vi "test14-Interrupt_Event.vi"(8 "error in (no error)":errorcluster, 11 "TestCase in":refnum<class "testcase-CSMGlobalLog.lvclass">) -> (0 "error out":errorcluster, 3 "TestCase out":refnum<class "testcase-CSMGlobalLog.lvclass">)   [LabVIEW 2017, in "testcase-CSMGlobalLog.lvclass"]
uses:
  testcase-CSMGlobalLog.lvclass
  testcase-CSMGlobalLog.lvclass/testcase-CSMGlobalLog.ctl
  src/user.lib/_NEVSTOP/Communicable State Machine(CSM)/_Support/Typedef/_CSM_GlobalLog_MSG.ctl
  src/user.lib/_NEVSTOP/Communicable State Machine(CSM)/_Support/Typedef/_CSM_Response Source Message.ctl
  src/user.lib/_NEVSTOP/Communicable State Machine(CSM)/_Support/Typedef/_CSM_GlobalLog_MSG_TYPE.ctl
  c0dc643a-0362-49fc-99f4-5251266ba5a0.vi
  src/user.lib/_NEVSTOP/Communicable State Machine(CSM)/_Support/GlobalEvent/GEvt-Generate with Rule Check.vi
  src/user.lib/_NEVSTOP/Communicable State Machine(CSM)/AdvanceAPI/CSM - Convert Error to Argument.vi
  src/user.lib/_NEVSTOP/Communicable State Machine(CSM)/AdvanceAPI/CSM - Make String Arguments Safe.vi
  src/user.lib/_NEVSTOP/Communicable State Machine(CSM)/AdvanceAPI/CSM - Keywords.vi
  src/user.lib/_NEVSTOP/Communicable State Machine(CSM)/_Support/GlobalEvent/Cache-GEvt Refs.vi
  src/user.lib/_NEVSTOP/Communicable State Machine(CSM)/_Support/GlobalEvent/LogFilter/LogFilter - Check.vi
  src/user.lib/_NEVSTOP/Communicable State Machine(CSM)/_Support/GlobalEvent/LogFilter/LogFilter.lvclass
  <vilib>/addons/_JKI Toolkits/VI Tester/TestCase.llb/TestCase.lvclass
  src/user.lib/_NEVSTOP/Communicable State Machine(CSM)/Communicable State Machine.lvlib
  C:/Program Files (x86)/National Instruments/LabVIEW 2017/vi.lib/addons/_JKI Toolkits/VI Tester/TestCase.llb/TestCase.lvclass
panel:
  out "String cache each loop":string
  out "error out 2":errorcluster
  out "Timed out":bool[](array[boolean])
  out "LoopCount":i32
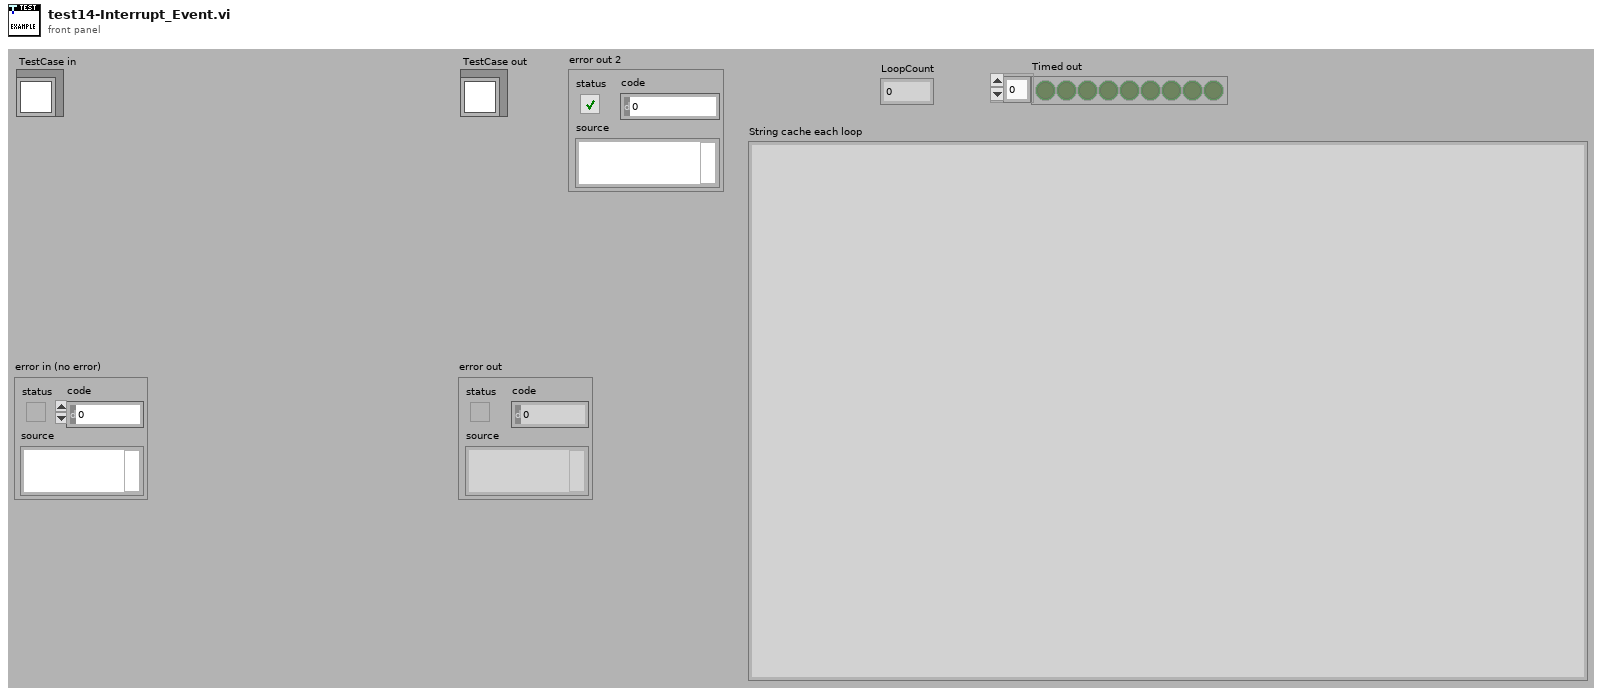
[diagram p1: front panel]
types:
  T1 = typedef "Communicable State Machine.lvlib/_CSM_GlobalLog_MSG.ctl" = cluster{"Name (\"\" to Use UUID)":string, "Current State":string, "Arguments":string, "Source Message":T2, "Source Module":string, "Complete(T)/Start(F)":bool, "LogType":T3, "Time Stamp":timestamp}
  T2 = typedef "Communicable State Machine.lvlib/_CSM_Response Source Message.ctl" = cluster{"‘State":string, "’Arguments":string, "’Error":errorcluster}
  T3 = typedef "Communicable State Machine.lvlib/_CSM_GlobalLog_MSG_TYPE.ctl" = enum16{"User Log", "State Change", "Status", "Interrupt", "Register", "Unregister", "Error Log", "Module Created", "Module Destroyed", "Async Message", "No-Rep Async Message", "Sync Message"}
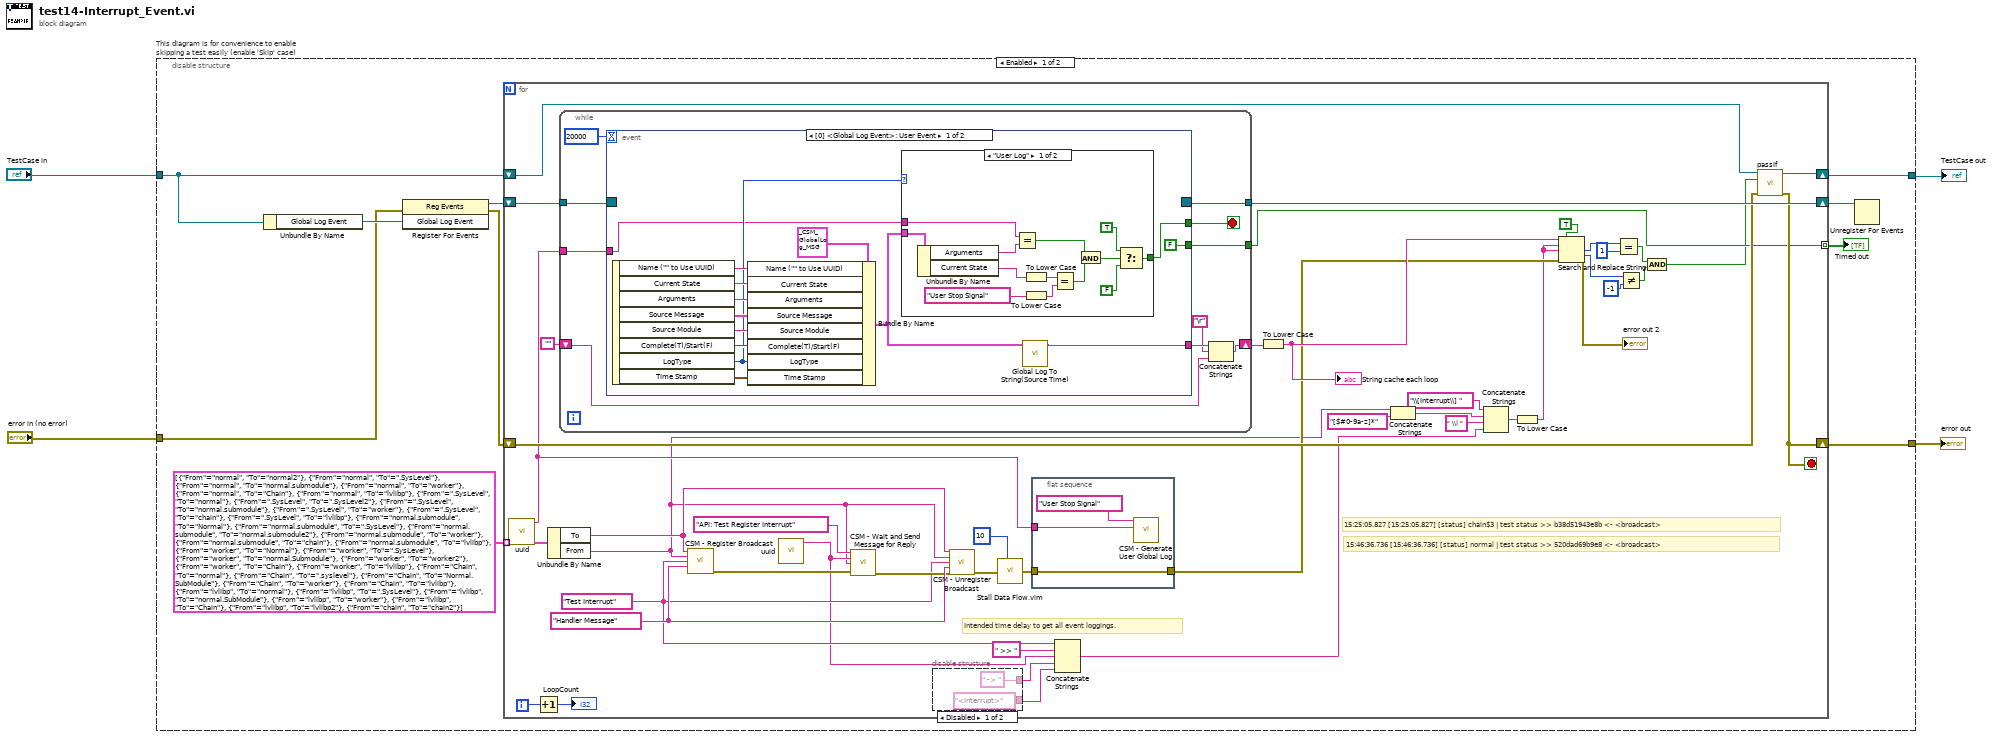
[diagram p0: block diagram]
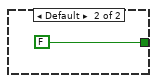
[diagram p3: hidden frame]
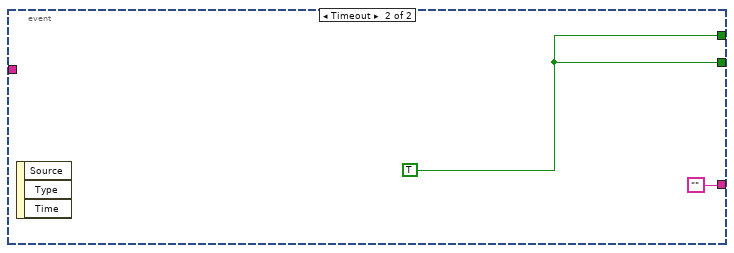
[diagram p4: hidden frame]
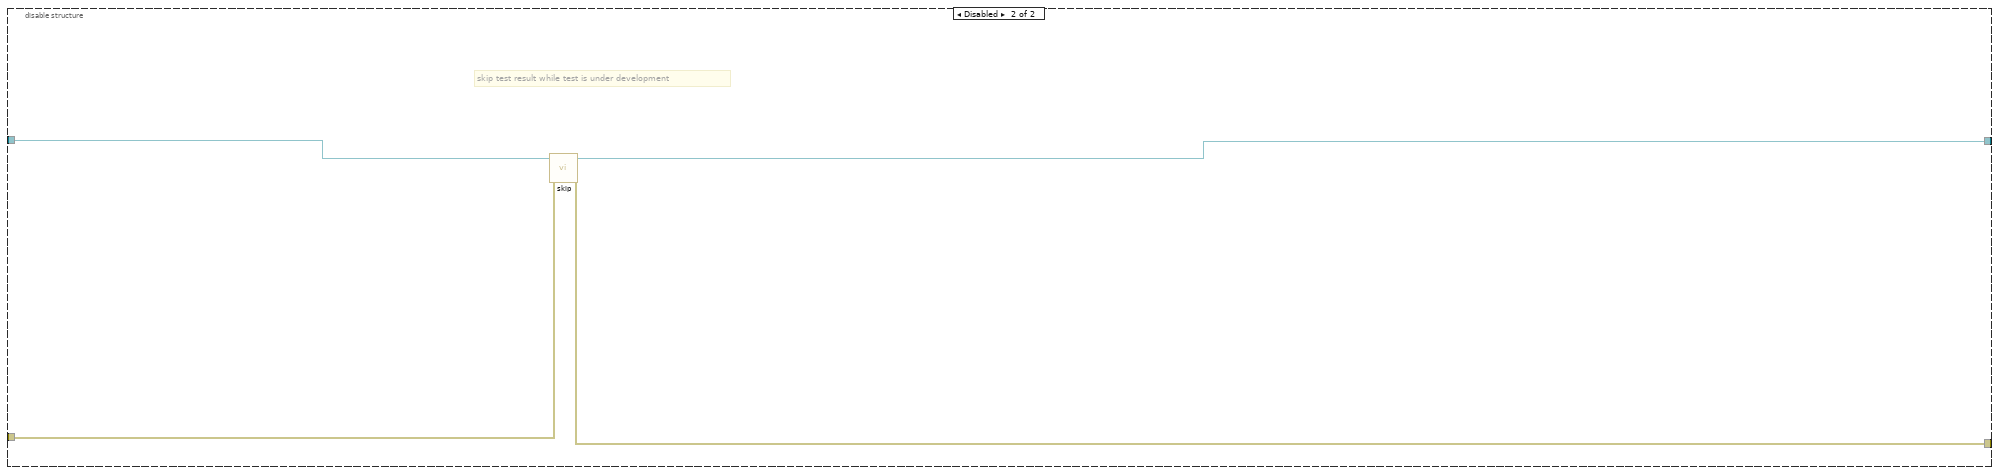
[diagram p5: hidden frame]
diagram:
  n1 = disable-structure "This diagram is for convenience to enable skipping a test easily (enable 'Skip' case)" shown="Enabled" {
    disable-tunnel: "TestCase in" -> [w9 w108]
    disable-tunnel: [w8 w106] -> w1
    disable-tunnel: [w7 w107] -> w3
    disable-tunnel: "error in (no error)" -> [w13 w105]
    frame Enabled {
      n2 = Unbundle By Name(w9) -> ("Global Log Event"=w14:refnum<user-event>)
      n3 = register-events(error in=w13, w14) -> (reference out=w12:refnum<event-registration>, error out=w10:errorcluster)  [unwired: 1 in]
      n4 = for {
        shift-right: [w58] -> w11
        shift-left: w12 -> [w59]
        shift-right: [w54] -> w7
        shift-left: w10 -> [w56]
        tunnel: cluster{"From":string, "To":string}[] [{"From"="normal", "To"="normal2"}, {"From"="normal", "To"=".SysLevel"}, {"From"="normal", "To"="normal.submodule"}, {"From"="normal", "To"="worker"}, {"From"="normal", "To"="Chain"}, {"From"="normal", "To"="lvlibp"}, {"From"=".SysLevel", "To"="normal"}, {"From"=".SysLevel", "To"=".SysLevel2"}, {"From"=".SysLevel", "To"="normal.submodule"}, {"From"=".SysLevel", "To"="worker"}, {"From"=".SysLevel", "To"="chain"}, {"From"=".SysLevel", "To"="lvlibp"}, {"From"="normal.submodule", "To"="Normal"}, {"From"="normal.submodule", "To"=".SysLevel"}, {"From"="normal.submodule", "To"="normal.submodule2"}, {"From"="normal.submodule", "To"="worker"}, {"From"="normal.submodule", "To"="chain"}, {"From"="normal.submodule", "To"="lvlibp"}, {"From"="worker", "To"="Normal"}, {"From"="worker", "To"=".SysLevel"}, {"From"="worker", "To"="normal.Submodule"}, {"From"="worker", "To"="worker2"}, {"From"="worker", "To"="Chain"}, {"From"="worker", "To"="lvlibp"}, {"From"="Chain", "To"="normal"}, {"From"="Chain", "To"=".syslevel"}, {"From"="Chain", "To"="Normal.SubModule"}, {"From"="Chain", "To"="worker"}, {"From"="Chain", "To"="lvlibp"}, {"From"="lvlibp", "To"="normal"}, {"From"="lvlibp", "To"=".SysLevel"}, {"From"="lvlibp", "To"="normal.SubModule"}, {"From"="lvlibp", "To"="worker"}, {"From"="lvlibp", "To"="Chain"}, {"From"="lvlibp", "To"="lvlibp2"}, {"From"="chain", "To"="chain2"}] -> [w31] mode=indexing
        shift-right: [w57] -> w8
        shift-left: w9 -> [w53]
        tunnel: [w37] -> w5 mode=indexing
        i -> [w42]
        stop <- w54 stop-if-true
        w36 = "Handler Message" ("API (If \"\", Same as Trigger)")
        w27 = "Test Interrupt" ("Trigger")
        # "15:46:36.736 [15:46:36.736] [status] normal | test status >> 520dad69b9e8 <- <broadcast>"
        # "15:25:05.827 [15:25:05.827] [status] chain$3 | test status >> b38d51943e8b <- <broadcast>"
        # "Intended time delay to get all event loggings."
        n5 = call "uuid.vi"() -> ("UUID"=w43:string)  [unwired: 11 in]
        n6 = Increment(x=w42) -> (x+1=→"LoopCount":i32)
        n7 = Unbundle By Name(w31) -> ("To"=w18:string, "From"=w17:string)
        n8 = while {
          tunnel: w59 -> [w74]
          tunnel: [w73] -> w58
          shift-right: [w65] -> w38
          shift-left: "" -> [w68]
          tunnel: w43 -> [w70]
          tunnel: [w69] -> w37
          stop <- w72 stop-if-true
          n9 = event shown="[0] <Global Log Event>: User Event" {
            selector: w74 -> [_ _]
            dyn-events: [_ _] -> w73
            timeout: 20000 -> [_ _]
            tunnel: [w75 ""] -> w67
            tunnel: [w77 w104] -> w72
            tunnel: w70 -> [w78 _]
            tunnel: [FALSE ("Stop") w104] -> w69
            event User Event {
              n10 = event-data() -> ("Name (\"\" to Use UUID)"=w87:string, "Current State"=w86:string, "Arguments"=w85:string, "Source Message"=w84:T2, "Source Module"=w83:string, "Complete(T)/Start(F)"=w82:bool, "LogType"=w79:T3, "Time Stamp"=w81:timestamp)  [unwired: 1 in]
              n11 = Bundle By Name(cluster=T1 {"Name (\"\" to Use UUID)"="", "Current State"="", "Arguments"="", "Source Message"={"‘State"="", "’Arguments"="", "’Error"={"status"=FALSE, "code"=0, "source"=""}}, "Source Module"="", "Complete(T)/Start(F)"=FALSE, "LogType"=enum."State Change", "Time Stamp"=timestamp(0 s since 1904-01-01)} ("Cross CSM Data"), "Name (\"\" to Use UUID)"=w87, "Current State"=w86, "Arguments"=w85, "Source Message"=w84, "Source Module"=w83, "Complete(T)/Start(F)"=w82, "LogType"=w79, "Time Stamp"=w81) -> (w76:T1)
              n12 = case shown="\"User Log\"" w79 {
                tunnel: w76 -> [w101 _]
                tunnel: w78 -> [w100 _]
                tunnel: [w89 FALSE] -> w77
                frame "User Log" {
                  n13 = Unbundle By Name(w101) -> ("Arguments"=w99:string, "Current State"=w98:string)
                  n14 = Equal?(x=w100, y=w99) -> (x = y?=w93:bool)
                  n15 = To Lower Case(string=w98) -> (all lower case string=w97:string)
                  n16 = To Lower Case(string="User Stop Signal" ("Log")) -> (all lower case string=w95:string)
                  n17 = Equal?(x=w97, y=w95) -> (x = y?=w94:bool)
                  n18 = And(x=w93, y=w94) -> (x .and. y?=w92:bool)
                  n19 = Select(t=TRUE, s=w92, f=FALSE) -> (s? t:f=w89:bool)
                }
                frame Default {
                }
              }
              n20 = call "Global Log To String(Source Time).vi"("Log"=w76) -> ("Log String"=w75:string)  [unwired: 9 in]
            }
            event Timeout {
              w104 = TRUE ("Stop")
              n21 = event-data() -> ()  [unwired: 1 in, 3 out]
            }
          }
          n22 = Concatenate Strings(w67, "\r", w68) -> (w65:string)
        }
        n23 = call "CSM - Register Broadcast.vi"("CSM Name(Empty for Broadcast Event)"=w18, "Source CSM Name (* as Default)"=w17, "Trigger"=w27, "API (If \"\", Same as Trigger)"=w36) -> ("error out"=w33:errorcluster)  [unwired: 10 in, 1 out]
        n24 = call "uuid.vi"() -> ("UUID"=w26:string)  [unwired: 11 in]
        n25 = call "CSM - Wait and Send Message for Reply.vi"("State"="API: Test Register Interrupt", "Arguments (\"\")"=w26, "Target Module"=w17, "Error In (No Error)"=w33) -> ("error out"=w34:errorcluster)  [unwired: 9 in, 2 out]
        n26 = disable-structure shown="Disabled" {
          disable-tunnel: [" -> " ("string") _] -> w29
          disable-tunnel: ["<interrupt>" ("search string") _] -> w28
          frame Disabled {
          }
          frame Enabled {
          }
        }
        n27 = call "CSM - Unregister Broadcast.vi"("CSM Name(Empty for Broadcast Event)"=w18, "Source CSM Name (* as Default)"=w17, "Trigger"=w27, "API (\"*\" as Default)"=w36, "Error In"=w34) -> ("error out"=w32:errorcluster)  [unwired: 9 in, 1 out]
        n28 = call "Stall Data Flow.vim"("value in"=w32, "milliseconds to wait"=u32 10) -> ("value out"=w44:errorcluster)  [unwired: 1 out]
        n29 = flat-sequence {
          tunnel: w43 -> [w63]
          tunnel: w44 -> [w62]
          tunnel: [w62] -> w39
          frame #0 {
            n30 = call "CSM - Generate User Global Log.vi"("Arguments"=w63, "Log"="User Stop Signal") -> ()  [unwired: 9 in, 1 out]
          }
        }
        n31 = Concatenate Strings(w27, " >> " ("string"), w26, w29, w28) -> (w16:string)
        n32 = To Lower Case(string=w38) -> (all lower case string=w40:string)
        "String cache each loop" <- w40
        n33 = Concatenate Strings(w17, "[$#0-9a-z]*" ("string")) -> (w19:string)
        n34 = Concatenate Strings("\\[Interrupt\\] " ("regular expression"), w19, " \\| " ("string"), w16) -> (w22:string)
        n35 = To Lower Case(string=w22) -> (all lower case string=w15:string)
        n36 = Search and Replace String(replace all?=TRUE ("replace all? (F)"), input string=w40, search string=w15, replace string=w15, error in=w39) -> (number of replacements=w49:i32, offset past replacement=w50:i32, error out=→"error out 2":errorcluster)  [unwired: 3 in, 1 out]
        n37 = Equal?(x=w49, y=1) -> (x = y?=w51:bool)
        n38 = Not Equal?(x=w50, y=-1) -> (x != y?=w52:bool)
        n39 = And(x=w51, y=w52) -> (x .and. y?=w25:bool)
        n40 = call-dynamic "passIf.vi"("error in (no error)"=w56, "pass"=w25, "TestCase in"=w53) -> ("error out"=w54:errorcluster, "TestCase out"=w57:refnum<class "testcase-CSMGlobalLog.lvclass">)  [unwired: 7 in]
      }
      "Timed out" <- w5
      n41 = Unregister For Events(event registration refnum=w11) -> ()  [unwired: 1 in, 1 out]
    }
    frame Disabled {
      # "skip test result while test is under development"
      n42 = call <vilib>:"skip.vi"("error in (no error)"=w105, "TestCase in"=w108) -> ("error out"=w107:errorcluster, "TestCase out"=w106:refnum<class "testcase-CSMGlobalLog.lvclass">)  [unwired: 8 in]
    }
  }
  "error out" <- w3
  "TestCase out" <- w1
